vi "RPM2DutyCycle.vi"(1 "Speed":dbl) -> (0 "Duty Cycle":dbl)   [LabVIEW 2016]
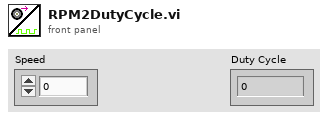
[diagram p1: front panel]
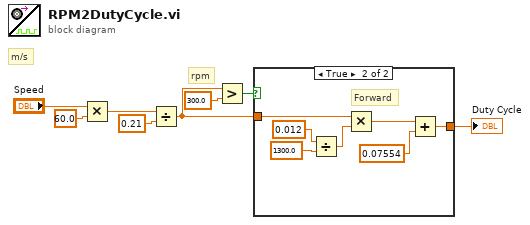
[diagram p0: block diagram]
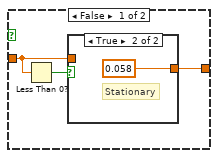
[diagram p2: hidden frame]
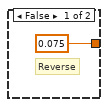
[diagram p3: hidden frame]
diagram:
  # "rpm"
  # "m/s"
  n1 = Multiply(x="Speed", y=60.0) -> (x*y=w3:dbl)
  n2 = Divide(x=w3, y=0.21) -> (x/y=w1:dbl)
  n3 = Greater?(x=w1, y=300.0) -> (0:w8:bool)
  n4 = case shown="True" w8 {
    tunnel: w1 -> [w9 w15]
    tunnel: [w10 w14] -> w7
    frame False {
      n5 = Less Than 0?(x=w9) -> (x < 0?=w11:bool)
      n6 = case shown="True" w11 {
        tunnel: [0.075 0.058] -> w10
        tunnel: w9 -> [_ _]
        frame False {
          # "Reverse"
        }
        frame True {
          # "Stationary"
        }
      }
    }
    frame True {
      # "Forward"
      n7 = Divide(x=0.012, y=1300.0) -> (x/y=w20:dbl)
      n8 = Multiply(x=w15, y=w20) -> (x*y=w19:dbl)
      n9 = Add(x=w19, y=0.07554) -> (x+y=w14:dbl)
    }
  }
  "Duty Cycle" <- w7
